vi "FTW-Test-Socket-Stress-RouterShutdown.vi"() -> (0 "Test Result":errorcluster)   [LabVIEW 2014]
panel:
  out "Endpoints":string[](array[string])
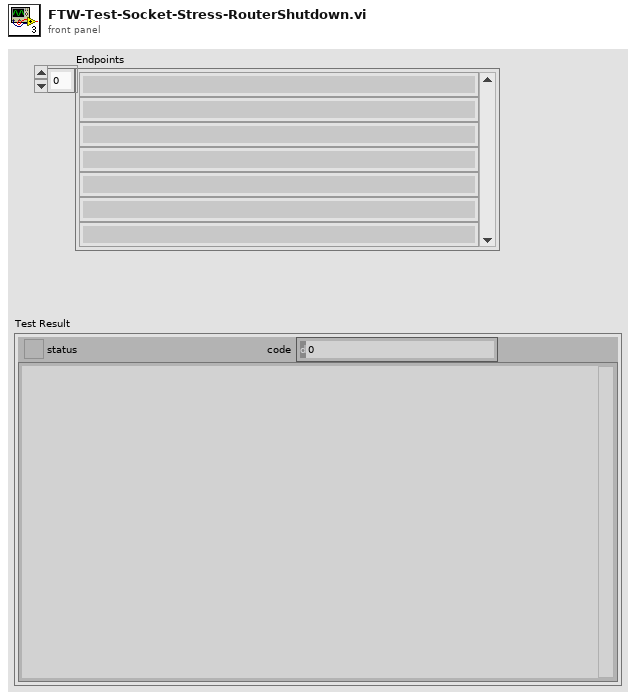
[diagram p1: front panel]
types:
  T1 = cluster{"[0]":refnum<event-registration>, "[1]":refnum<event-registration>, "[2]":refnum<event-registration>, "[3]":refnum<event-registration>, "[4]":refnum<event-registration>, "[5]":refnum<event-registration>, "[6]":refnum<event-registration>, "[7]":refnum<event-registration>, "[8]":refnum<event-registration>, "[9]":refnum<event-registration>, "[10]":refnum<event-registration>, "[11]":refnum<event-registration>, "[12]":refnum<event-registration>, "[13]":refnum<event-registration>, "[14]":refnum<event-registration>, "[15]":refnum<event-registration>, "[16]":refnum<event-registration>, "[17]":refnum<event-registration>, "[18]":refnum<event-registration>, "[19]":refnum<event-registration>}
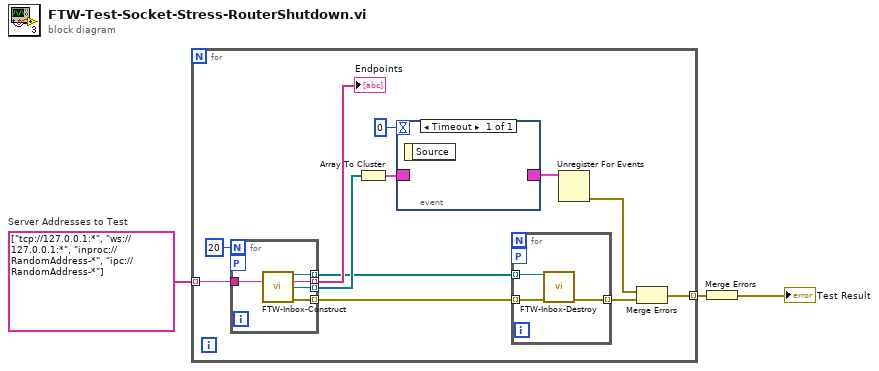
[diagram p0: block diagram]
diagram:
  w3 = string[] ["tcp://127.0.0.1:*", "ws://127.0.0.1:*", "inproc://RandomAddress-*", "ipc://RandomAddress-*"]  # Server Addresses to Test
  n1 = for {
    tunnel: [w10] -> w1 mode=indexing
    tunnel: w3 -> [w4] mode=indexing
    n2 = for {
      N: 20 -> [_]
      tunnel: [w23] -> w7 mode=indexing
      tunnel: [w22] -> w8 mode=indexing
      tunnel: [w21] -> w14 mode=indexing
      tunnel: [w20] -> w12 mode=indexing
      tunnel: w4 -> [w19]
      workers-P: _ -> [_]
      n3 = call "FTW-Inbox-Construct.vi"("Primary Inbox Address"=w19) -> ("FTW Router"=w23:refnum<data-value>, "Resolved Primary Inbox Address"=w22:string, "Incoming Request"=w21:refnum<event-registration>, "error out"=w20:errorcluster)  [unwired: 11 in]
    }
    "Endpoints" <- w8
    n4 = Array To Cluster(array=w14) -> (cluster=w5:T1)
    n5 = event shown="[0] Timeout" {
      selector: w5 -> [_]
      dyn-events: [_] -> w13
      timeout: 0 -> [_]
      event Timeout {
        n6 = event-data() -> ()  [unwired: 1 in, 1 out]
      }
    }
    n7 = for {
      tunnel: w7 -> [w18] mode=indexing
      tunnel: w12 -> [w17] mode=indexing
      tunnel: [w16] -> w11 mode=indexing
      workers-P: _ -> [_]
      n8 = call "FTW-Inbox-Destroy.vi"("FTW Router"=w18, "error in"=w17) -> ("error out"=w16:errorcluster)  [unwired: 13 in]
    }
    n9 = Unregister For Events(event registration refnum=w13) -> (error out=w6:errorcluster)  [unwired: 1 in]
    n10 = Merge Errors(w6, w11) -> (w10:errorcluster)
  }
  n11 = Merge Errors(w1) -> (→"Test Result":errorcluster)
